vi "xcorr_running.vi"(4 "Array 5":fxp<+,1,1>[](array[numeric]), 5 "Element":fxp<+/-,16,16>, 6 "Array 6":fxp<+,1,1>[](array[numeric]), 7 "Element 2":fxp<+/-,16,16>, 9 "Array 7":fxp<+,1,1>[](array[numeric]), 10 "Array 4":fxp<+,1,1>[](array[numeric]), 11 "Element 3":fxp<+/-,16,16>) -> (1 "Array":fxp<+,1,1>[](array[numeric]), 2 "Array 2":fxp<+,1,1>[](array[numeric]), 3 "Array 3":fxp<+,1,1>[](array[numeric]))   [LabVIEW 2015]
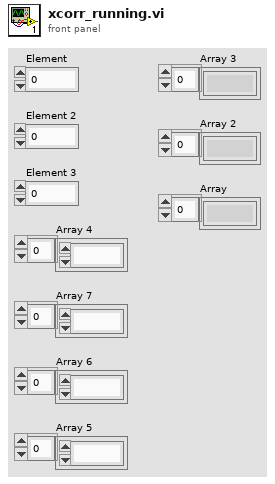
[diagram p1: front panel]
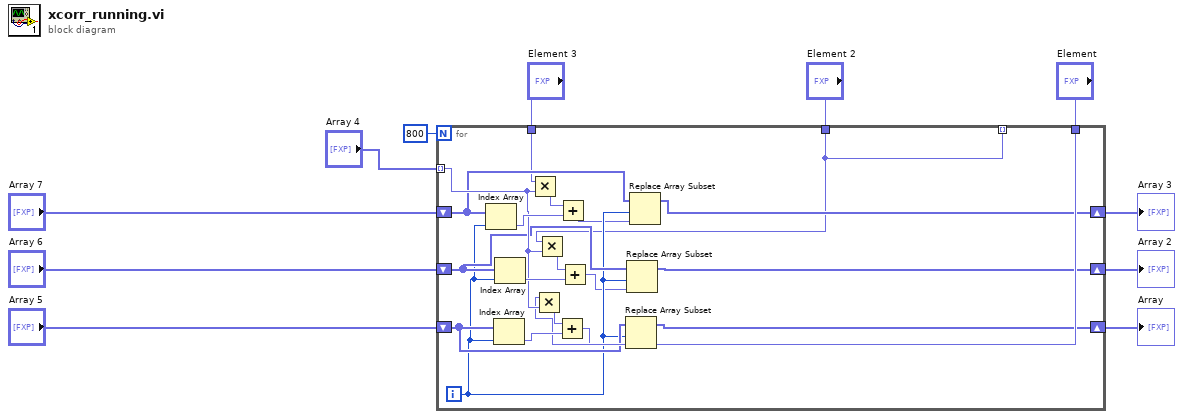
[diagram p0: block diagram]
diagram:
  n1 = for {
    N: 800 -> [_]
    shift-right: [w16] -> w9
    shift-left: "Array 7" -> [w23]
    shift-right: [w15] -> w10
    shift-left: "Array 6" -> [w22]
    shift-right: [w14] -> w11
    shift-left: "Array 5" -> [w21]
    tunnel: "Array 4" -> [w28] mode=indexing
    tunnel: "Element 3" -> [w13]
    tunnel: "Element 2" -> [w12]
    tunnel: "Element" -> [w27]
    tunnel: [w12] -> _ mode=indexing
    i -> [w20]
    n2 = Index Array(array=w23, index=w20) -> (element=w29:fxp<+,1,1>)
    n3 = Index Array(array=w21, index=w20) -> (element=w31:fxp<+,1,1>)
    n4 = Index Array(array=w22, index=w20) -> (element=w30:fxp<+,1,1>)
    n5 = Multiply(x=w13, y=w28) -> (x*y=w24:fxp<+,1,1>)
    n6 = Multiply(x=w27, y=w28) -> (x*y=w26:fxp<+,1,1>)
    n7 = Multiply(x=w12, y=w28) -> (x*y=w25:fxp<+,1,1>)
    n8 = Add(x=w26, y=w31) -> (x+y=w17:fxp<+,1,1>)
    n9 = Add(x=w24, y=w29) -> (x+y=w18:fxp<+,1,1>)
    n10 = Add(x=w25, y=w30) -> (x+y=w19:fxp<+,1,1>)
    n11 = Replace Array Subset(array=w21, new element=w17, index=w20) -> (w14:fxp<+,1,1>[])
    n12 = Replace Array Subset(array=w22, new element=w19, index=w20) -> (w15:fxp<+,1,1>[])
    n13 = Replace Array Subset(array=w23, new element=w18, index=w20) -> (w16:fxp<+,1,1>[])
  }
  "Array" <- w11
  "Array 2" <- w10
  "Array 3" <- w9
